vi "absortion_load.vi"(11 "all rows":dbl[][](array[numeric])) -> (3 "curva atenuation":cluster{"Energia":dbl[], "coeficiente":dbl[]})   [LabVIEW 2021]
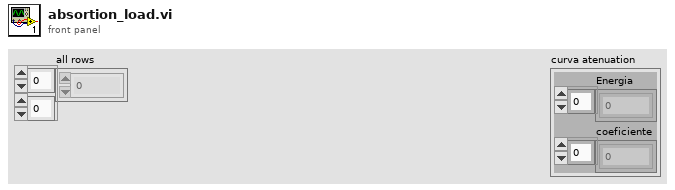
[diagram p1: front panel]
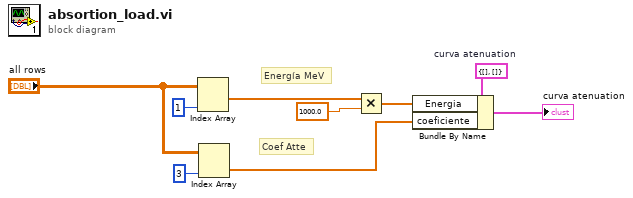
[diagram p0: block diagram]
diagram:
  w8 = cluster{"Energia":dbl[], "coeficiente":dbl[]} {"Energia"=[], "coeficiente"=[]}  # curva atenuation
  # "Coef Atte"
  # "Energía MeV"
  n1 = Index Array(array="all rows", index (col)=1 ("disabled index (col)")) -> (element=w3:dbl[])  [unwired: 1 in]
  n2 = Index Array(array="all rows", index (col)=3 ("disabled index (col)")) -> (element=w7:dbl[])  [unwired: 1 in]
  n3 = Multiply(x=w3, y=1000.0) -> (x*y=w1:dbl[])
  n4 = Bundle By Name(cluster=w8, "Energia"=w1, "coeficiente"=w7) -> (→"curva atenuation":cluster{"Energia":dbl[], "coeficiente":dbl[]})
